vi "Create All Message Queues.vi"(8 "error in":errorcluster) -> (0 "error out":errorcluster, 3 "Queues":T1)   [LabVIEW 2015, in "Message Queue.lvlib"]
doc: "Creates and initializes message queues"
uses:
  Message Queue.lvlib
  All Message Queues.ctl
  Message Cluster.ctl
  Enqueue Message (Single).vi
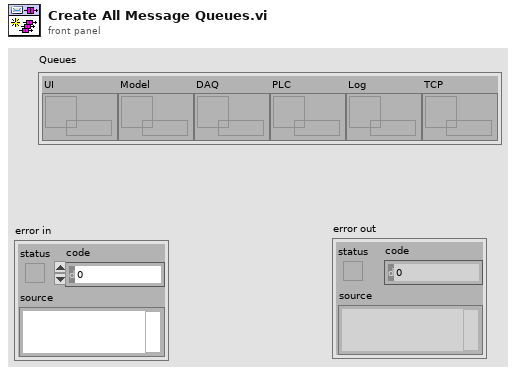
[diagram p1: front panel]
types:
  T1 = typedef "Message Queue.lvlib/All Message Queues.ctl" = cluster{"UI":refnum<queue>, "Model":refnum<queue>, "DAQ":refnum<queue>, "PLC":refnum<queue>, "Log":refnum<queue>, "TCP":refnum<queue>}
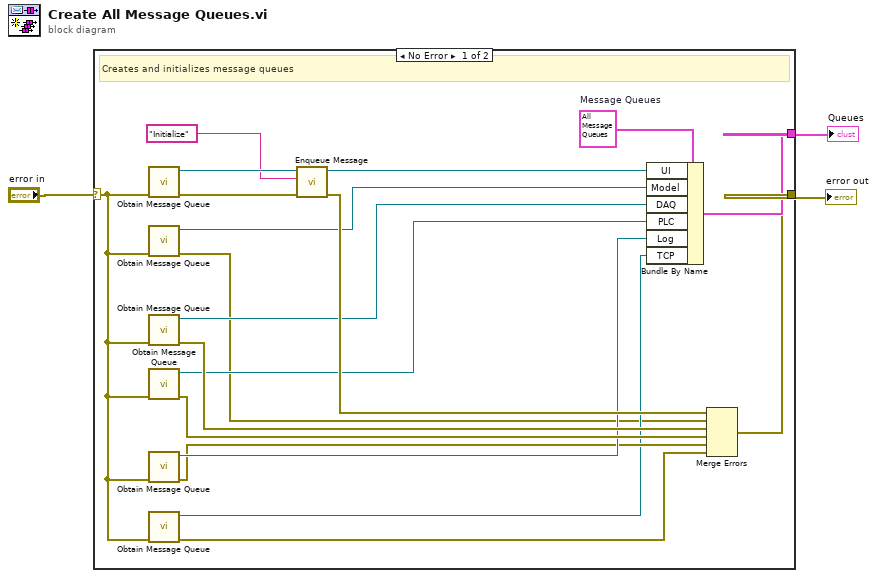
[diagram p0: block diagram]
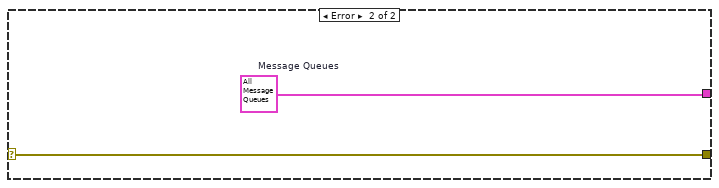
[diagram p2: hidden frame]
diagram:
  n1 = case shown="No Error" "error in" {
    selector: "error in" -> [w15 w24]
    tunnel: [w16 w24] -> w3
    tunnel: [w21 w23] -> w2
    frame No Error {
      w22 = T1 {"UI"=refnum, "Model"=refnum, "DAQ"=refnum, "PLC"=refnum, "Log"=refnum, "TCP"=refnum}  # Message Queues
      # "Creates and initializes message queues"
      n2 = call "Obtain Message Queue.vi"("error in (no error)"=w15) -> ("error out"=w20:errorcluster, "Message Queue"=w19:refnum<queue>)  [unwired: 9 in]
      n3 = call "Obtain Message Queue.vi"("error in (no error)"=w15) -> ("error out"=w5:errorcluster, "Message Queue"=w4:refnum<queue>)  [unwired: 9 in]
      n4 = call "Obtain Message Queue.vi"("error in (no error)"=w15) -> ("error out"=w12:errorcluster, "Message Queue"=w13:refnum<queue>)  [unwired: 9 in]
      n5 = call "Obtain Message Queue.vi"("error in (no error)"=w15) -> ("error out"=w10:errorcluster, "Message Queue"=w11:refnum<queue>)  [unwired: 9 in]
      n6 = call "Obtain Message Queue.vi"("error in (no error)"=w15) -> ("error out"=w8:errorcluster, "Message Queue"=w9:refnum<queue>)  [unwired: 9 in]
      n7 = call "Obtain Message Queue.vi"("error in (no error)"=w15) -> ("error out"=w6:errorcluster, "Message Queue"=w7:refnum<queue>)  [unwired: 9 in]
      n8 = call-poly "Enqueue Message.vi"("error in (no error)"=w20, "Message"="Initialize", "Message Queue"=w19) -> ("error out"=w17:errorcluster, "dup Message Queue"=w18:refnum<queue>)  [unwired: 7 in]
      n9 = Bundle By Name(cluster=w22, "UI"=w18, "Model"=w4, "DAQ"=w13, "PLC"=w11, "Log"=w9, "TCP"=w7) -> (w21:T1)
      n10 = Merge Errors(w17, w5, w12, w10, w8, w6) -> (w16:errorcluster)
    }
    frame Error {
      w23 = T1 {"UI"=refnum, "Model"=refnum, "DAQ"=refnum, "PLC"=refnum, "Log"=refnum, "TCP"=refnum}  # Message Queues
    }
  }
  "Queues" <- w2
  "error out" <- w3
